vi "KE622x -- 2182 -A Query.vi"(0 "622x Resource In":refnum<visa-resource-name>, 1 "Check For SCPI Errors? (T)":bool=TRUE, 7 "2182-A Write String":string, 9 "Max Num Bytes To Read (256)":u32=256, 11 "error in (no error)":errorcluster) -> (4 "622x Resource Out (dupl)":refnum<visa-resource-name>, 8 "2182-A Reponse String":string, 15 "error out":errorcluster)   [LabVIEW 2019, in "Keithley 622x.lvlib"]
uses:
  Keithley 622x.lvlib
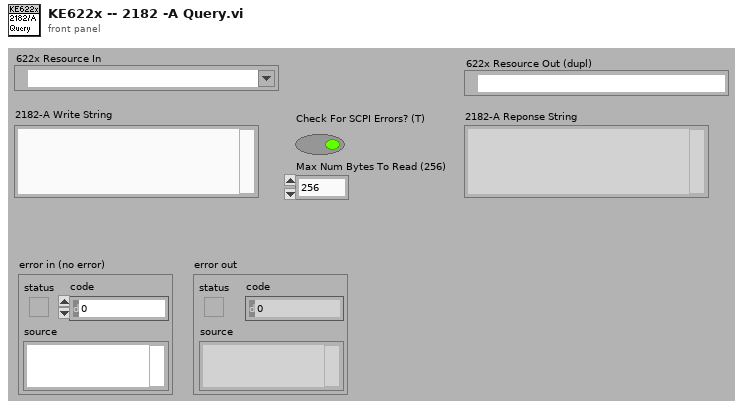
[diagram p1: front panel]
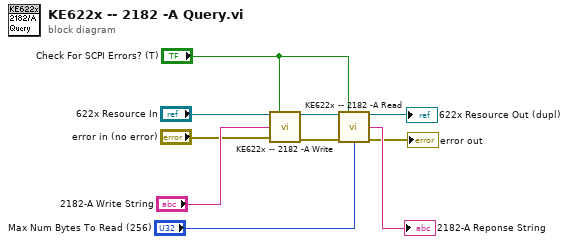
[diagram p0: block diagram]
diagram:
  n1 = call "KE622x -- 2182 -A Write.vi"("Resource In"="622x Resource In", "Check For SCPI Errors? (T)"="Check For SCPI Errors? (T)", "2182-A Write String"="2182-A Write String", "error in (no error)"="error in (no error)") -> ("Resource Out (dupl)"=w7:refnum<visa-resource-name>, "error out"=w6:errorcluster)  [unwired: 10 in]
  n2 = call "KE622x -- 2182 -A Read.vi"("622x Resource In"=w7, "Check For SCPI Errors? (T)"="Check For SCPI Errors? (T)", "error in (no error)"=w6, "Max Num Bytes To Read (256)"="Max Num Bytes To Read (256)") -> ("622x Resource Out (dupl)"=→"622x Resource Out (dupl)":refnum<visa-resource-name>, "2182-A Reponse String"=→"2182-A Reponse String":string, "error out"=→"error out":errorcluster)  [unwired: 9 in]
